vi "LorentzianFunc.vi"(7 "B":dbl, 8 "d":dbl, 9 "A":dbl, 10 "x0":dbl, 11 "X":dbl) -> (3 "B+A/[1+(X-X0)^2 / d^2]":dbl)   [LabVIEW 2015]
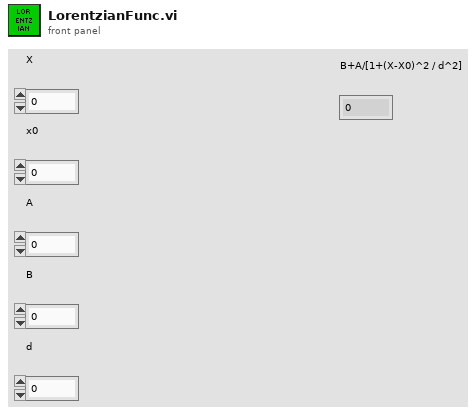
[diagram p1: front panel]
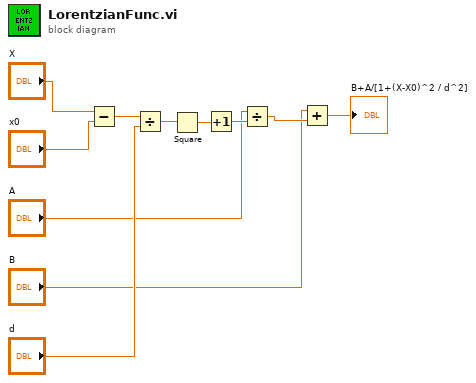
[diagram p0: block diagram]
diagram:
  n1 = Subtract(x="X", y="x0") -> (x-y=w9:dbl)
  n2 = Divide(x=w9, y="d") -> (x/y=w7:dbl)
  n3 = Square(x=w7) -> (x^2=w6:dbl)
  n4 = Increment(x=w6) -> (x+1=w5:dbl)
  n5 = Divide(x="A", y=w5) -> (x/y=w3:dbl)
  n6 = Add(x="B", y=w3) -> (x+y=→"B+A/[1+(X-X0)^2 / d^2]":dbl)
